vi "teleportBallErForce.vi"(8 "error in (no error)":errorcluster, 10 "ballReplacement":T1, 11 "Communication in":refnum<class "Communication.lvclass">) -> (0 "error out":errorcluster, 2 "teleportBallArray":u8[](array[numeric]), 3 "Communication out":refnum<class "Communication.lvclass">)   [LabVIEW 2023, in "Communication.lvclass"]
uses:
  Communication.lvclass
  grSim Packet Command UDP Test Folder/grSim/grSim_BallReplacement.ctl
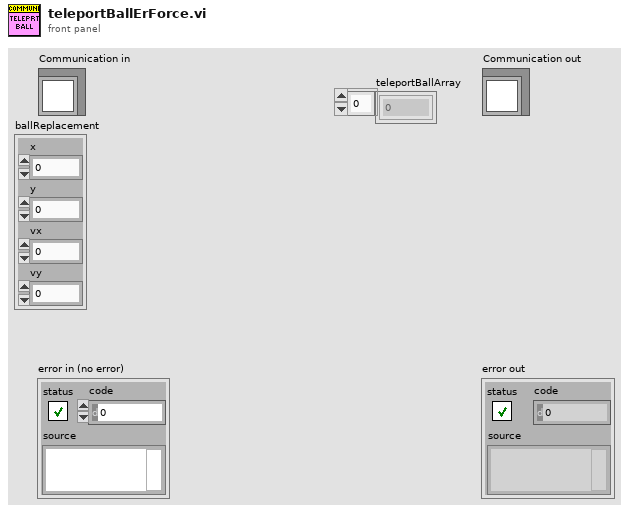
[diagram p1: front panel]
types:
  T1 = typedef "grSim_BallReplacement.ctl" = cluster{"x":dbl, "y":dbl, "vx":dbl, "vy":dbl}
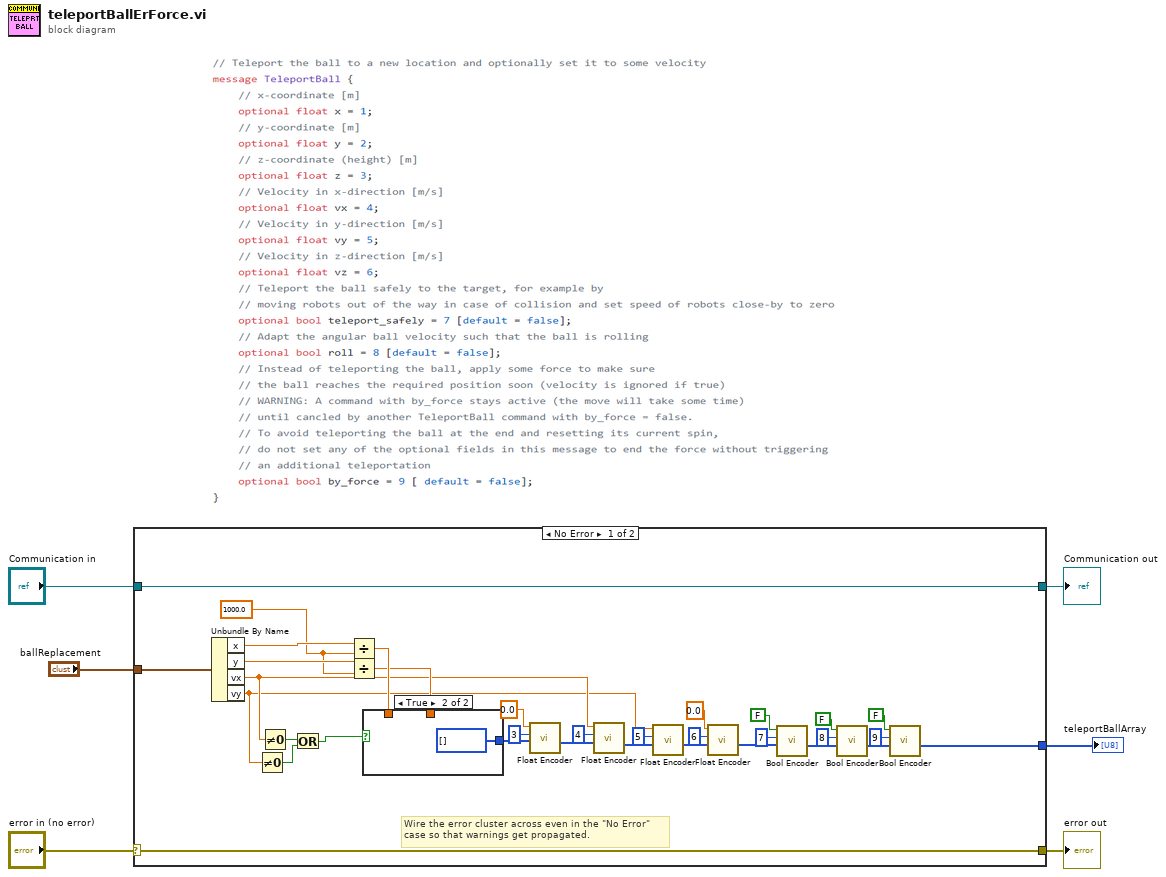
[diagram p0: block diagram]
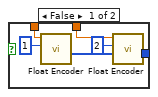
[diagram p2: hidden frame]
diagram:
  n1 = case shown="No Error" "error in (no error)" {
    selector: "error in (no error)" -> [w38 w48]
    tunnel: [w38 w48] -> w5
    tunnel: [w39 w47] -> w3
    tunnel: "Communication in" -> [w39 w47]
    tunnel: [w18 _] -> w2
    tunnel: "ballReplacement" -> [w17 _]
    frame No Error {
      w13 = 1000.0
      # "Wire the error cluster across even in the \"No Error\"\ncase so that warnings get propagated."
      n2 = Unbundle By Name(w17) -> ("x"=w16:dbl, "y"=w14:dbl, "vx"=w11:dbl, "vy"=w8:dbl)
      n3 = Not Equal To 0?(x=w8) -> (x != 0?=w9:bool)
      n4 = Not Equal To 0?(x=w11) -> (x != 0?=w10:bool)
      n5 = Or(x=w10, y=w9) -> (x .or. y?=w7:bool)
      n6 = Divide(x=w16, y=w13) -> (x/y=w15:dbl)
      n7 = Divide(x=w14, y=w13) -> (x/y=w12:dbl)
      n8 = case shown="True" w7 {
        tunnel: [w45 u8[] [] ("Array")] -> w37
        tunnel: w15 -> [w44 _]
        tunnel: w12 -> [w43 _]
        frame False {
          n9 = call "Float Encoder.vi"("Key"=u32 1, "Value"=w44) -> ("Array"=w41:u8[])  [unwired: 9 in]
          n10 = call "Float Encoder.vi"("Array In"=w41, "Key"=u32 2, "Value"=w43) -> ("Array"=w45:u8[])  [unwired: 8 in]
        }
        frame True {
        }
      }
      n11 = call "Float Encoder.vi"("Array In"=w37, "Key"=u32 3, "Value"=sgl 0.0) -> ("Array"=w34:u8[])  [unwired: 8 in]
      n12 = call "Float Encoder.vi"("Array In"=w34, "Key"=u32 4, "Value"=w11) -> ("Array"=w32:u8[])  [unwired: 8 in]
      n13 = call "Float Encoder.vi"("Array In"=w32, "Key"=u32 5, "Value"=w8) -> ("Array"=w30:u8[])  [unwired: 8 in]
      n14 = call "Float Encoder.vi"("Array In"=w30, "Key"=u32 6, "Value"=sgl 0.0) -> ("Array"=w27:u8[])  [unwired: 8 in]
      n15 = call "Bool Encoder.vi"("Array In"=w27, "Key"=u32 7, "Value"=FALSE) -> ("Array"=w24:u8[])  [unwired: 8 in]
      n16 = call "Bool Encoder.vi"("Array In"=w24, "Key"=u32 8, "Value"=FALSE) -> ("Array"=w21:u8[])  [unwired: 8 in]
      n17 = call "Bool Encoder.vi"("Array In"=w21, "Key"=u32 9, "Value"=FALSE) -> ("Array"=w18:u8[])  [unwired: 8 in]
    }
    frame Error {
    }
  }
  "error out" <- w5
  "Communication out" <- w3
  "teleportBallArray" <- w2
